vi "Test PUBLISH packet.vi"(8 "error in (no error)":errorcluster) -> (0 "error out":errorcluster)   [LabVIEW 2013]
uses:
  source/Control Packets/ControlPacket/QualityOfService -- enum.ctl
  source/Control Packets/PUBLISH/PUBLISH.lvclass
  source/Control Packets/ControlPacket/ControlPacket.lvclass/ControlPacket.ctl
  source/Control Packets/ControlPacket/ControlPacket.lvclass
  <vilib>/addons/_JKI Toolkits/Caraya/classes/Test/Test.lvclass
  <vilib>/addons/_JKI Toolkits/Caraya/classes/Assert/Assert.lvclass
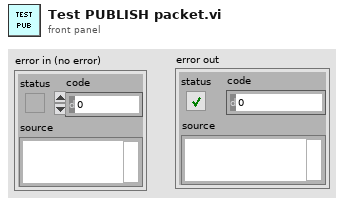
[diagram p1: front panel]
types:
  T1 = typedef "MQTT_Control_Packets.lvlib/ControlPacket.lvclass/QualityOfService -- enum.ctl" = enum16{"0 (At Most Once)", "1 (At Least Once)", "2 (Exactly Once)"}
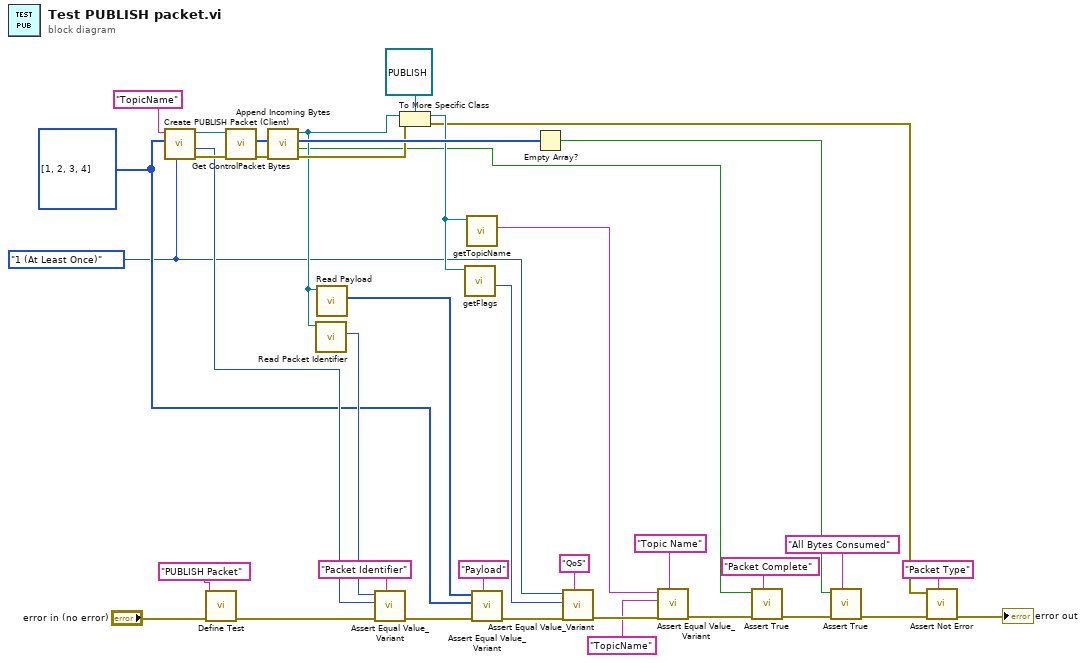
[diagram p0: block diagram]
diagram:
  w13 = u8[] [1, 2, 3, 4] ("Payload")
  w6 = QualityOfService_--_enum."1 (At Least Once)" ("QoS")
  n1 = call "Create PUBLISH Packet (Client).vi"("QoS"=w6, "Payload"=w13, "Topic Name"="TopicName") -> ("error out"=w33:errorcluster, "Packet ID"=w16:u16, "PUBLISH"=w34:refnum<class "PUBLISH.lvclass">)  [unwired: 6 in]
  n2 = call <vilib>:"Define Test.vi"("error in (no error)"="error in (no error)", "Label (VI Title)"="PUBLISH Packet") -> ("error out"=w23:errorcluster)  [unwired: 9 in]
  n3 = call "Get ControlPacket Bytes.vi"("error in (no error)"=w33, "ControlPacket"=w34) -> ("error out"=w36:errorcluster, "Bytes Stream"=w38:u8[])  [unwired: 6 in, 2 out]
  n4 = call "Append Incoming Bytes.vi"("error in (no error)"=w36, "Incoming Packets"=w38) -> ("error out"=w35:errorcluster, "Complete Packet"=w18:bool, "Remaining Packets"=w37:u8[], "ControlPacket"=w30:refnum<class "ControlPacket.lvclass">)  [unwired: 6 in]
  n5 = call "Read Packet Identifier.vi"("ControlPacket in"=w30) -> ("Packet Identifier"=w17:u16)  [unwired: 9 in, 1 out]
  n6 = call "Read Payload.vi"("ControlPacket in"=w30) -> ("Payload"=w12:u8[])  [unwired: 9 in, 1 out]
  n7 = call <vilib>:"Assert Equal Value_Variant.vi"("Label"="Packet Identifier" ("Label (VI Title)"), "error in (no error)"=w23, "Y"=w16, "X"=w17) -> ("error out"=w14:errorcluster)  [unwired: 7 in]
  n8 = To More Specific Class(target class=refnum<class "PUBLISH.lvclass"> refnum ("MQTT_Control_Packets.lvlib:PUBLISH.lvclass"), reference=w30, error in=w35) -> (specific class reference=w31:refnum<class "PUBLISH.lvclass">, error out=w20:errorcluster)
  n9 = call-dynamic "getFlags.vi"("PUBLISH in"=w31) -> ("QoS"=w7:T1)  [unwired: 7 in, 3 out]
  n10 = call "getTopicName.vi"("PUBLISH in"=w31) -> ("Topic"=w5:string)  [unwired: 8 in, 2 out]
  n11 = call <vilib>:"Assert Equal Value_Variant.vi"("Label"="Payload" ("Label (VI Title)"), "error in (no error)"=w14, "Y"=w13, "X"=w12) -> ("error out"=w11:errorcluster)  [unwired: 7 in]
  n12 = Empty Array?(array=w37) -> (empty?=w19:bool)
  n13 = call <vilib>:"Assert Equal Value_Variant.vi"("Label"="QoS" ("Label (VI Title)"), "error in (no error)"=w11, "Y"=w7, "X"=w6) -> ("error out"=w10:errorcluster)  [unwired: 7 in]
  n14 = call <vilib>:"Assert Equal Value_Variant.vi"("Label"="Topic Name" ("Label (VI Title)"), "error in (no error)"=w10, "Y"="TopicName" ("Topic Name"), "X"=w5) -> ("error out"=w1:errorcluster)  [unwired: 7 in]
  n15 = call <vilib>:"Assert True.vi"("Label"="Packet Complete" ("Label (VI Title)"), "error in (no error)"=w1, "True?"=w18) -> ("error out"=w24:errorcluster)  [unwired: 8 in]
  n16 = call <vilib>:"Assert True.vi"("Label"="All Bytes Consumed" ("Label (VI Title)"), "error in (no error)"=w24, "True?"=w19) -> ("error out"=w3:errorcluster)  [unwired: 8 in]
  n17 = call <vilib>:"Assert Not Error.vi"("Label"="Packet Type" ("Label (VI Title)"), "error in (no error)"=w3, "Not Error?"=w20) -> ("error out"=→"error out":errorcluster)  [unwired: 8 in]
